vi "State_Init_Data Map.vi"(8 "error in (no error)":errorcluster, 9 "Data":T1[](array[typedef]), 10 "Channel":string[](array[string]), 11 "MB Slave in":refnum<class "MB Slave Simulator Base.lvclass">) -> (0 "error out":errorcluster, 1 "CVT Size":i32, 2 "Debug Message":string, 3 "MB Slave out":refnum<class "MB Slave Simulator Base.lvclass">)   [LabVIEW 2021, in "MB Slave Simulator Base.lvclass"]
uses:
  MB Slave Simulator Base.lvclass
  C:/Program Files (x86)/National Instruments/LabVIEW 2021/user.lib/S2 Labs/Module Framework/Modules/Base/Module.lvclass
  C:/Program Files (x86)/National Instruments/LabVIEW 2021/user.lib/S2 Labs/Module Framework/Modules/Modbus/Modbus Slave Base/Modbus Slave Base.lvclass
  <userlib>/S2 Labs/CVT Toolkit/TypeDefs/Data Cluster.ctl
  <userlib>/S2 Labs/CVT Toolkit/CVT.lvclass/CVT.ctl
  <userlib>/S2 Labs/Module Framework/Modules/Modbus/Modbus Slave Base/Modbus Slave Base.lvclass/Modbus Slave Base.ctl
  <userlib>/S2 Labs/Module Framework/Modules/Base/Module.lvclass/Module.ctl
  888c1b1f-915e-4a14-9e5b-313d3a67477f.vi
  a51cec90-f002-4bcc-8fa1-84661e774747.vi
  <userlib>/S2 Labs/Module Framework/Modules/Modbus/Modbus Slave Base/Read MB Ref.vi
  888c1b1f-915e-4a14-9e5b-313d3a67477f.vi/1553f4ce-967c-4f57-a913-5f155bf4374d.vi
  a51cec90-f002-4bcc-8fa1-84661e774747.vi/71b19a30-41bb-452f-8775-2cd3e07414b9.vi
  <userlib>/S2 Labs/Module Framework/Modules/Base/Read Module CVT.vi
  <userlib>/S2 Labs/CVT Toolkit/Read CVT DVR.vi
  <userlib>/S2 Labs/CVT Toolkit/Variant Functions/Write Reserved Attributes.vi
  <userlib>/S2 Labs/CVT Toolkit/Variant Functions/Write Alias Attribute.vi
  <userlib>/S2 Labs/CVT Toolkit/Variant Functions/Write Unit Attribute.vi
  <userlib>/S2 Labs/CVT Toolkit/Variant Functions/Write Type Attribute.vi
  <userlib>/S2 Labs/CVT Toolkit/Variant Functions/Write Parms Attribute.vi
  <userlib>/S2 Labs/Module Framework/Modules/Base/Get Module CVT Ref.vi
  <userlib>/S2 Labs/Module Framework/Modules/Base/Trigger Logging Write.vi
  <userlib>/S2 Labs/Module Framework/Modules/Modbus/Modbus Slave Base/Modbus Slave Base.lvclass
  <userlib>/S2 Labs/Modbus Toolkit/Slave/S2L Modbus Slave.lvclass
  <userlib>/S2 Labs/CVT Toolkit/CVT.lvclass
  MB Slave Simulator Base.lvclass/MB Slave Simulator Base.ctl
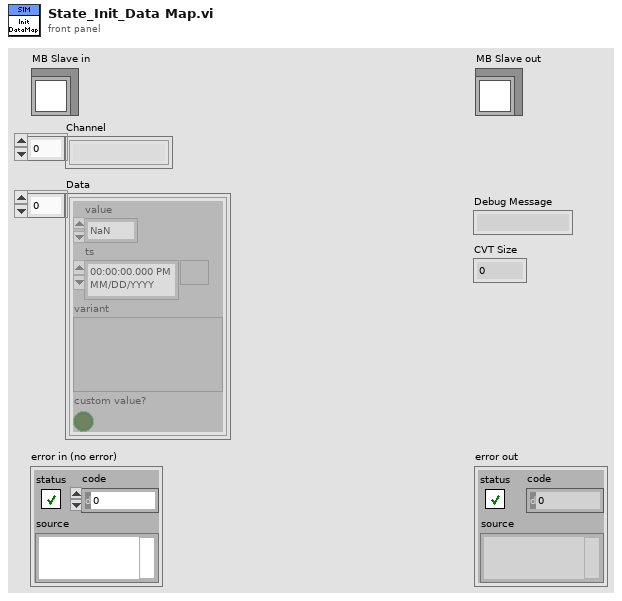
[diagram p1: front panel]
types:
  T1 = typedef "CVT.lvclass/Data Cluster.ctl" = cluster{"value":dbl, "ts":timestamp, "variant":variant, "custom value?":bool}
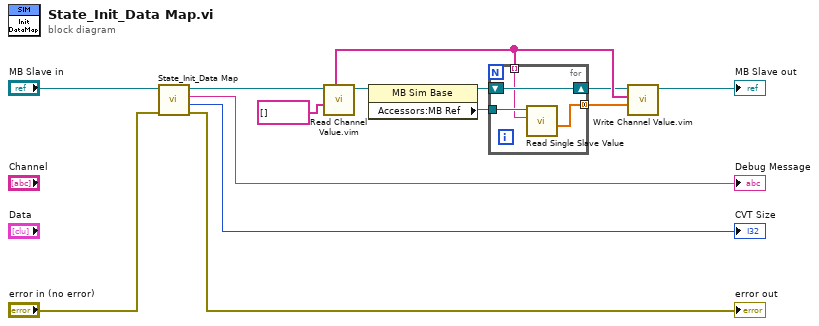
[diagram p0: block diagram]
diagram:
  n1 = call-parent "State_Init_Data Map.vi"("error in (no error)"="error in (no error)", "MB Slave in"="MB Slave in") -> ("error out"=→"error out":errorcluster, "CVT Size"=→"CVT Size":i32, "Debug Message"=→"Debug Message":string, "MB Slave out"=w8:refnum<class "MB Slave Simulator Base.lvclass">)  [unwired: 6 in]
  n2 = call "Read Channel Value.vim"("Channel Label(s)"=string[] [], "Module in"=w8) -> ("Module out"=w9:refnum<class "MB Slave Simulator Base.lvclass">, "Channel Labels*"=w13:string[])  [unwired: 3 in, 5 out]
  n3 = property class="MB Sim Base"(reference=w9) -> (reference out=w11:refnum<class "MB Slave Simulator Base.lvclass">, "Accessors:MB Ref"=w10:refnum<class "S2L Modbus Slave.lvclass">)  [unwired: 1 in, 1 out]
  n4 = for {
    tunnel: w10 -> [w18]
    shift-right: [w17] -> w12
    shift-left: w11 -> [w17]
    tunnel: w13 -> [w16] mode=indexing
    tunnel: [w15] -> w14 mode=concatenating
    n5 = call-dynamic "Read Single Slave Value.vi"("Label"=w16, "S2L Modbus Slave in"=w18) -> ("Value (s)"=w15:dbl[])  [unwired: 4 in, 5 out]
  }
  n6 = call "Write Channel Value.vim"("value"=w14, "Channel Label(s)"=w13, "Module in"=w12) -> ("Module out"=→"MB Slave out":refnum<class "MB Slave Simulator Base.lvclass">)  [unwired: 6 in, 2 out]
